vi "Send acquired data result msg.vi"(0 "Message Enqueuer in":refnum<class "Message Enqueuer.lvclass">, 1 "Data in Volts":i16[](array[numeric]), 3 "error in (no error)":errorcluster, 4 "Message Priority (Normal)":T1=enum."Normal") -> (7 "Message Enqueuer out":refnum<class "Message Enqueuer.lvclass">, 10 "error out":errorcluster)   [LabVIEW 2015, in "Acquired data result msg.lvclass"]
uses:
  Acquire data request message/Acquired data result msg.lvclass
  <vilib>/ActorFramework/Message Enqueuer/Message Priority.ctl
  <vilib>/ActorFramework/Message Enqueuer/Message Enqueuer.lvclass
  Acquire data request message/Acquired data result msg.lvclass/Acquired data result msg.ctl
  <vilib>/ActorFramework/Message Enqueuer/Message Enqueuer.lvclass/Message Enqueuer.ctl
  <vilib>/ActorFramework/Message Priority Queue/Priority Enqueue.vi
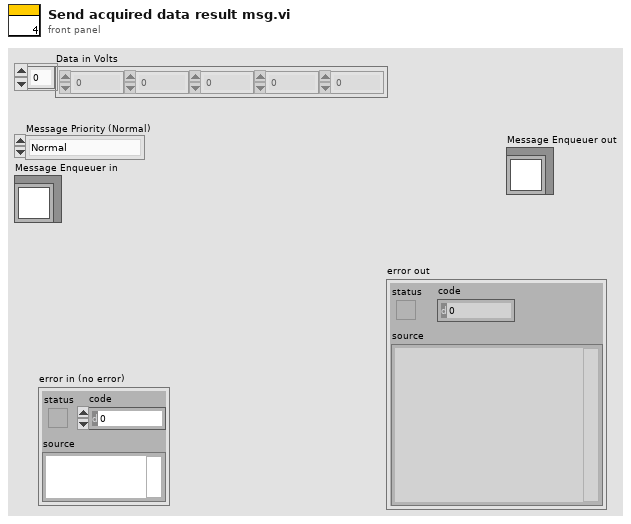
[diagram p1: front panel]
types:
  T1 = typedef "Actor Framework.lvlib/Message Enqueuer.lvclass/Message Priority.ctl" = enum16{"Low", "Normal", "High"}
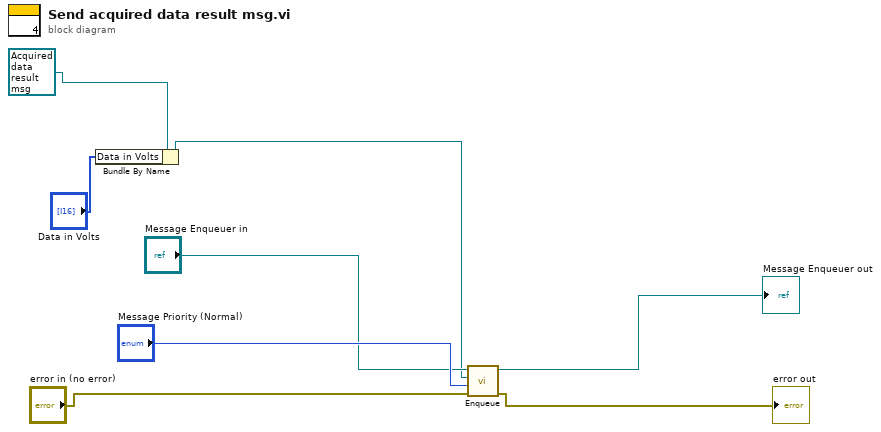
[diagram p0: block diagram]
diagram:
  n1 = Bundle By Name(cluster=refnum<class "Acquired data result msg.lvclass"> refnum ("Acquired data result msg.lvclass"), "Data in Volts"="Data in Volts") -> (w3:refnum<class "Acquired data result msg.lvclass">)
  n2 = call <vilib>:"Enqueue.vi"("error in (no error)"="error in (no error)", "Message Priority (Normal)"="Message Priority (Normal)", "Message"=w3, "Message Enqueuer in"="Message Enqueuer in") -> ("error out"=→"error out":errorcluster, "Message Enqueuer out"=→"Message Enqueuer out":refnum<class "Message Enqueuer.lvclass">)  [unwired: 6 in]
